vi "Add Cell.vi"(8 "error in":errorcluster, 10 "Cell Address":string, 11 "Row in":refnum<k24>) -> (0 "error out":errorcluster, 2 "Cell":refnum<k24>, 3 "Row out":refnum<k24>)   [LabVIEW 2019, in "Open Xml.lvlib"]
uses:
  Open Xml.lvlib
  D:/git/Open-Xml-LabVIEW/Source/DocumentFormat.OpenXml.dll
  DocumentFormat.OpenXml.dll
  D:/git/Open-Xml-LabVIEW/Source/DocumentFormat.OpenXml.Framework.dll
  DocumentFormat.OpenXml.Framework.dll
  D:/git/Open-Xml-LabVIEW/Source/OpenXmlGenericsWrapper.dll
  OpenXmlGenericsWrapper.dll
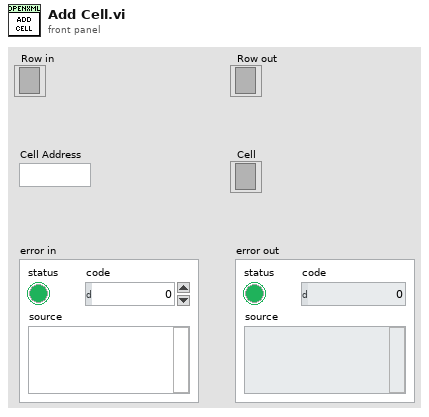
[diagram p1: front panel]
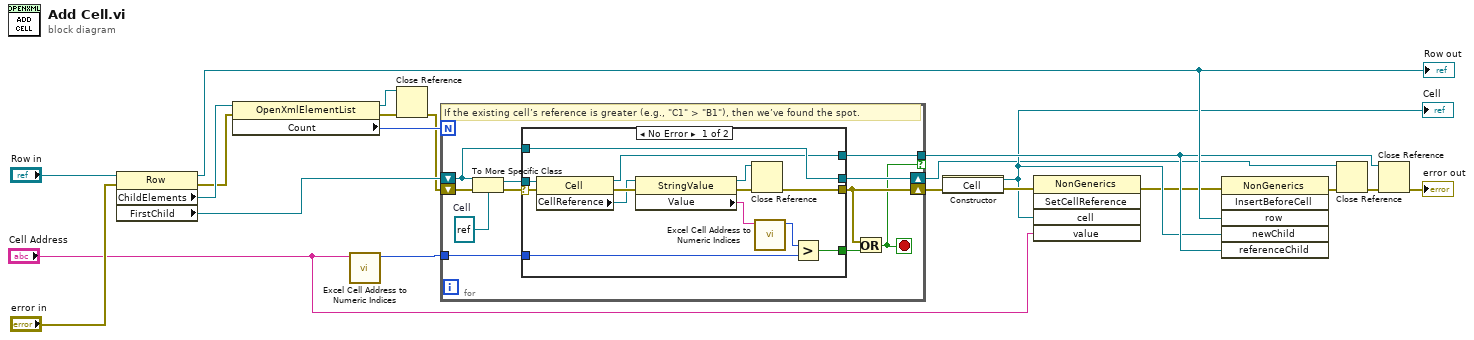
[diagram p0: block diagram]
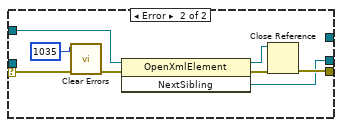
[diagram p2: hidden frame]
diagram:
  n1 = property class="Row"(reference="Row in", error in="error in") -> (reference out=w10:refnum<k24>, error out=w16:errorcluster, "ChildElements"=w20:refnum<k24>, "FirstChild"=w18:refnum<k24>)
  "Row out" <- w10
  n2 = property class="OpenXmlElementList"(reference=w20, error in=w16) -> (reference out=w11:refnum<k24>, error out=w17:errorcluster, "Count"=w19:i32)
  n3 = call "Excel Cell Address to Numeric Indices.vi"("Cell Name"="Cell Address") -> ("Column Number"=w15:i32)  [unwired: 9 in, 1 out]
  n4 = Close Reference(reference=w11, error in (no error)=w17) -> (error out=w12:errorcluster)
  n5 = for {
    N: w19 -> [_]
    tunnel: w15 -> [w26]
    shift-right: [w25] -> w1
    shift-left: w18 -> [w27]
    tunnel: [w24] -> w8 if=w23
    shift-right: [w29] -> w4
    shift-left: w12 -> [w30]
    stop <- w23 stop-if-true
    w31 = refnum<k24> refnum  # Cell
    # "If the existing cell’s reference is greater (e.g., \"C1\" > \"B1\"), then we’ve found the spot."
    n6 = To More Specific Class(target class=w31, reference=w27, error in=w30) -> (specific class reference=w28:refnum<k24>, error out=w32:errorcluster)
    n7 = case shown="No Error" w32 {
      selector: w32 -> [w45 w53]
      tunnel: [w34 w47] -> w29
      tunnel: w28 -> [w44 _]
      tunnel: w27 -> [w36 w50]
      tunnel: w26 -> [w40 _]
      tunnel: [w37 _] -> w22
      tunnel: [w36 w46] -> w25
      tunnel: [w35 _] -> w24
      frame No Error {
        n8 = property class="Cell"(reference=w44, error in=w45) -> (reference out=w35:refnum<k24>, error out=w43:errorcluster, "CellReference"=w42:refnum<k24>)
        n9 = property class="StringValue"(reference=w42, error in=w43) -> (reference out=w33:refnum<k24>, error out=w39:errorcluster, "Value"=w41:string)
        n10 = Close Reference(reference=w33, error in (no error)=w39) -> (error out=w34:errorcluster)
        n11 = call "Excel Cell Address to Numeric Indices.vi"("Cell Name"=w41) -> ("Column Number"=w38:i32)  [unwired: 9 in, 1 out]
        n12 = Greater?(x=w38, y=w40) -> (0:w37:bool)
      }
      frame Error {
        n13 = call <vilib>:"Clear Errors.vi"("error in (no error)"=w53, "specific error code to clear (0: all)"=1035) -> ("error out"=w51:errorcluster)  [unwired: 4 in, 1 out]
        n14 = invoke class="OpenXmlElement" method="NextSibling"(reference=w50, error in=w51) -> (reference out=w49:refnum<k24>, error out=w48:errorcluster, "NextSibling"=w46:refnum<k24>)  [unwired: 1 in]
        n15 = Close Reference(reference=w49, error in (no error)=w48) -> (error out=w47:errorcluster)
      }
    }
    n16 = Or(x=w29, y=w22) -> (x .or. y?=w23:bool)
  }
  n17 = constructor class="Cell"(error in=w4) -> (reference out=w5:refnum<k24>, error out=w14:errorcluster)  [unwired: 2 in, 1 out]
  "Cell" <- w5
  n18 = invoke class="NonGenerics" method="SetCellReference"(error in=w14, "cell"=w5, "value"="Cell Address") -> (error out=w3:errorcluster)  [unwired: 2 in, 4 out]
  n19 = invoke class="NonGenerics" method="InsertBeforeCell"(error in=w3, "row"=w10, "newChild"=w5, "referenceChild"=w8) -> (error out=w6:errorcluster)  [unwired: 2 in, 5 out]
  n20 = Close Reference(reference=w1, error in (no error)=w6) -> (error out=w2:errorcluster)
  n21 = Close Reference(reference=w8, error in (no error)=w2) -> (error out=→"error out":errorcluster)
